vi "Parse name to container.vi"(8 "error in":errorcluster, 10 "Create Unowned Container?":bool, 11 "Fully Qualified Name":string) -> (0 "error out":errorcluster, 3 "Container DGML Strings":string[](array[string]))   [LabVIEW 2018, in "DGML creation.lvlib"]
uses:
  DGML Creation/DGML creation.lvlib
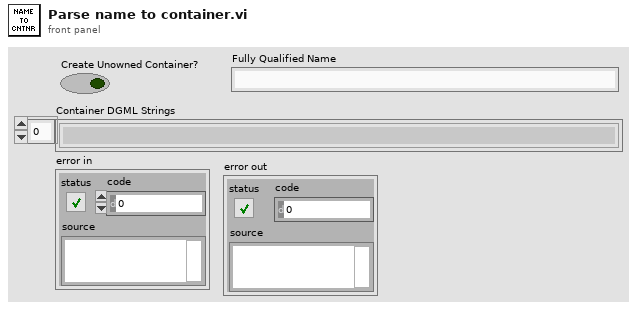
[diagram p1: front panel]
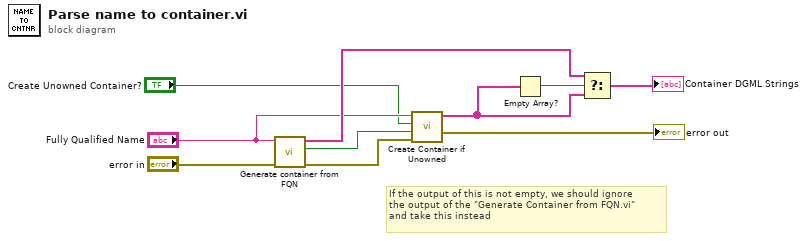
[diagram p0: block diagram]
diagram:
  # "If the output of this is not empty, we should ignore\nthe output of the \"Generate Container from FQN.vi\" \nand take this instead"
  n1 = call "Generate container from FQN.vi"("error in (no error)"="error in", "Fully Qualified Name"="Fully Qualified Name") -> ("error out"=w9:errorcluster, "Unowned?"=w4:bool, "DGML Strings"=w6:string[])  [unwired: 7 in]
  n2 = call "Create Container if Unowned.vi"("error in (no error)"=w9, "Item Is Unowned?"=w4, "Create Unowned Container?"="Create Unowned Container?", "Fully Qualified Name"="Fully Qualified Name") -> ("error out"=→"error out":errorcluster, "DGML Strings out"=w3:string[])  [unwired: 6 in]
  n3 = Empty Array?(array=w3) -> (empty?=w7:bool)
  n4 = Select(t=w6, s=w7, f=w3) -> (s? t:f=→"Container DGML Strings":string[])
